vi "Get Data Variant.vi"(8 "error in (no error)":errorcluster, 11 "Core Threads Configuration in":refnum<class "Thread Configuration.lvclass">) -> (0 "error out":errorcluster, 1 "data version":T1, 2 "data":variant, 3 "Core Threads Configuration out":refnum<class "Thread Configuration.lvclass">)   [LabVIEW 2017, in "DSF Core.lvlib" / "Thread Configuration.lvclass"]
uses:
  Thread Configuration.lvclass
  Typedefs/DSF Version Info.ctl
  Thread Configuration.lvclass/Thread Configuration.ctl
  DSF Core.lvlib
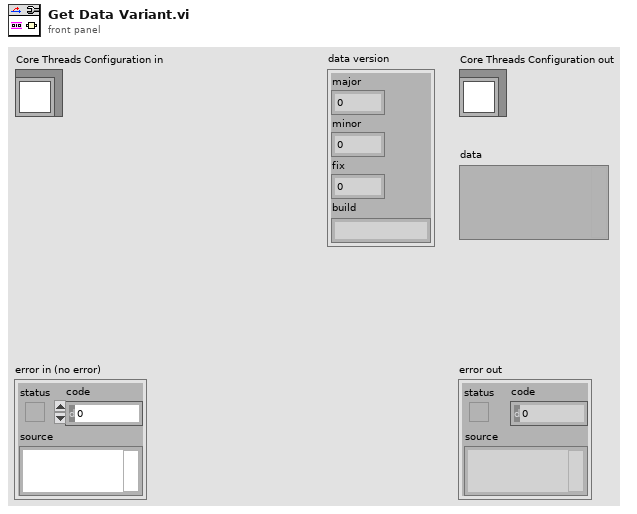
[diagram p1: front panel]
types:
  T1 = typedef "DSF Core.lvlib/DSF Version Info.ctl" = cluster{"major":u32, "minor":u32, "fix":u32, "build":string}
  T2 = typedef "DSF Core.lvlib/DSF Core Thread Configuration.ctl" = cluster{"processor":i32, "priority offset":i16}
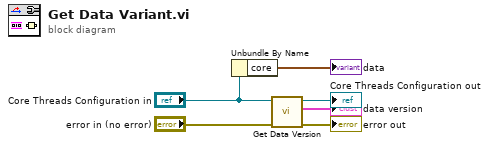
[diagram p0: block diagram]
diagram:
  n1 = Unbundle By Name("Core Threads Configuration in") -> ("core"=→"data":T2)
  n2 = call-dynamic "Get Data Version.vi"("error in (no error)"="error in (no error)", "Core Threads Configuration in"="Core Threads Configuration in") -> ("error out"=→"error out":errorcluster, "data version"=→"data version":T1, "Core Threads Configuration out"=→"Core Threads Configuration out":refnum<class "Thread Configuration.lvclass">)  [unwired: 7 in]
